vi "測試環境2.vi"() -> ()   [LabVIEW 2021]
panel:
  in  "停止":bool
  in  "輸入資料":dbl(slide) scale=0.0..100.0
  out "壓力計":dbl(xcontrol)
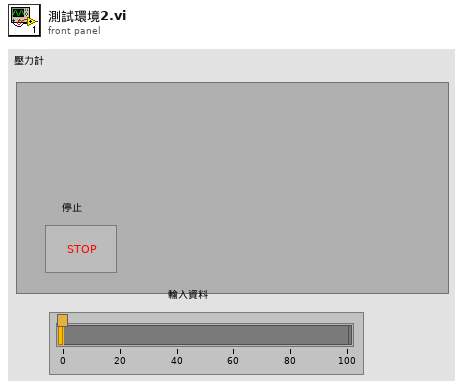
[diagram p1: front panel]
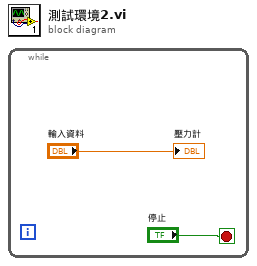
[diagram p0: block diagram]
diagram:
  n1 = while {
    stop <- "停止" stop-if-true
    "壓力計" <- "輸入資料"
  }
